vi "DeltaSingleRead.vi"() -> ()   [LabVIEW 2019]
uses:
  Global 2.vi
panel:
  out "Sample Temp [K]":dbl
  out "Delta Reading [Ohm]":dbl=1.19099581
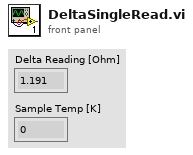
[diagram p1: front panel]
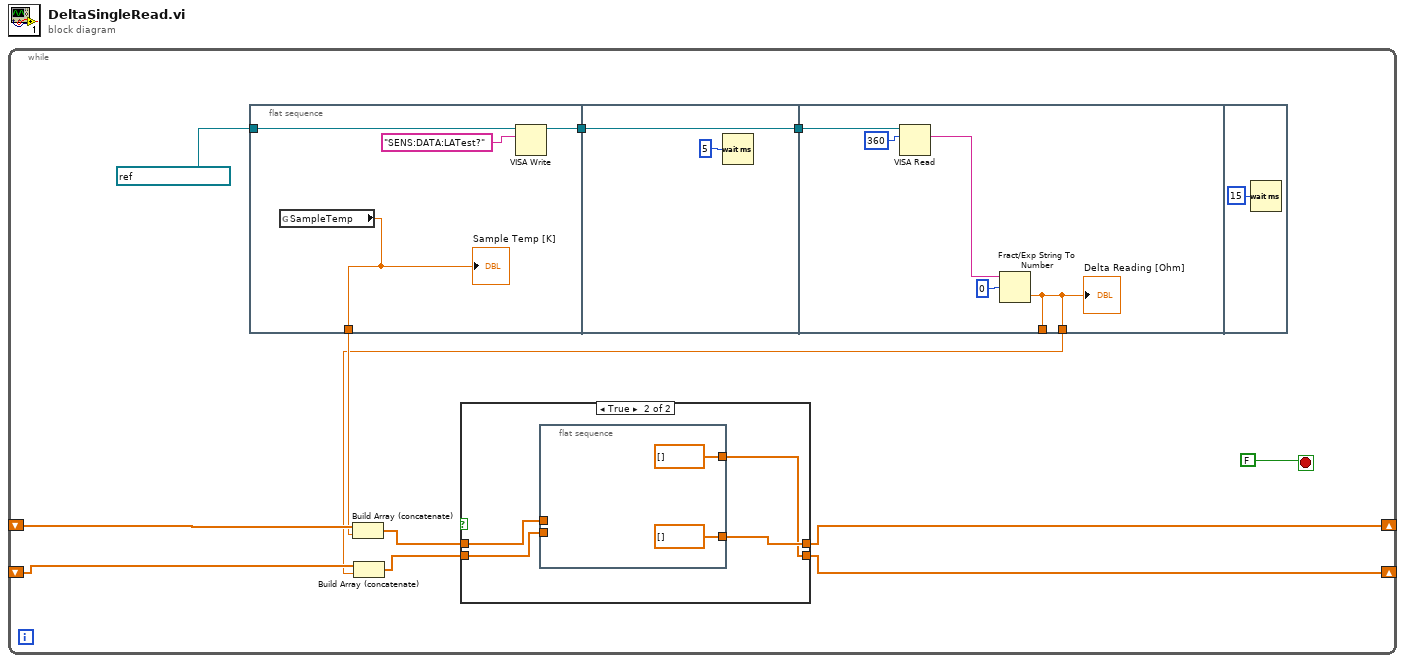
[diagram p0: block diagram]
diagram:
  n1 = while {
    shift-right: [w4] -> _
    shift-left: _ -> [w8]
    shift-right: [w1] -> _
    shift-left: _ -> [w6]
    stop <- FALSE stop-if-true
    n2 = flat-sequence {
      tunnel: [w23] -> w12
      tunnel: refnum<visa-resource-name> "GPIB1::20::INSTR" ("Keithley") -> [w22]
      tunnel: [w21] -> w3
      tunnel: [w25] -> w11
      tunnel: w12 -> [w25]
      tunnel: [w27] -> _
      tunnel: w11 -> [w28]
      tunnel: [w27] -> w2
      frame #0 {
        n3 = global read "Global 2.vi" "SampleTemp"() -> (w21:dbl)
        "Sample Temp [K]" <- w21
        n4 = VISA Write(VISA resource name=w22, write buffer="SENS:DATA:LATest?" ("write buffer 2")) -> (VISA resource name out=w23:refnum<visa-resource-name>)  [unwired: 1 in, 2 out]
      }
      frame #1 {
        n5 = Wait (ms)(milliseconds to wait=5) -> ()  [unwired: 1 out]
      }
      frame #2 {
        n6 = VISA Read(VISA resource name=w28, byte count=u32 360) -> (read buffer=w30:string)  [unwired: 1 in, 3 out]
        n7 = Fract/Exp String To Number(string=w30, offset=0) -> (number=w27:dbl)  [unwired: 3 out]
        "Delta Reading [Ohm]" <- w27
      }
      frame #3 {
        n8 = Wait (ms)(milliseconds to wait=15) -> ()  [unwired: 1 out]
      }
    }
    n9 = Build Array (concatenate)(w8, w3) -> (w7:dbl[])
    n10 = Build Array (concatenate)(w6, w2) -> (w5:dbl[])
    n11 = case shown="True" {
      selector: _ -> [_ _]
      tunnel: w7 -> [w14 w18]
      tunnel: [w14 w17] -> w4
      tunnel: w5 -> [w13 w16]
      tunnel: [w13 w15] -> w1
      frame False {
      }
      frame True {
        n12 = flat-sequence {
          tunnel: w18 -> [_]
          tunnel: w16 -> [_]
          tunnel: [dbl[] []] -> w15
          tunnel: [dbl[] []] -> w17
          frame #0 {
          }
        }
      }
    }
  }
